vi "Day 10 - Pipe Maze.vi"() -> ()   [LabVIEW 2020, in "AoC 2023.lvlib"]
uses:
  AoC 2023.lvlib
  3d240fc5-b77a-4919-ab2e-2db28b4f468f.vi
  3d240fc5-b77a-4919-ab2e-2db28b4f468f.vi/a6c839c9-92fd-4c27-961e-592a9f44c727.vi
  <vilib>/Analysis/geometry.llb/Point in Polygon.vi
  <vilib>/Analysis/geometry.llb/Point in Polygon (Scalar).vi
panel:
  in  "Tab Control":enum32{"GRID", "CHART"}(tab)
  out "GRID":string[][](array[string])
  out "XY Graph":cluster{"X":dbl, "Y":dbl}[](graph)
  in  "TIMEOUT":i32
  out "Puzzle Part-2 Answer":string
  out "Puzzle Answer":string
  in  "Puzzle Inputs":string[](array[string])=["7-F7-\n.FJ|7\nSJLL7\n|F--J\nLJ.LJ", "-L|F7\n7S-7|\nL|7||\n-L-J|\nL|-JF", "7-F7-\n.FJ|7\nSJLL7\n|F--J\nLJ.LJ", "...........\n.S-------7.\n.|F-----7|.\n.||.....||.\n.||.....||.\n.|L-7.F-J|.\n.|..|.|..|.\n.L--J.L--J.\n...........", ".F----7F7F7F7F-7....\n.|F--7||||||||FJ....\n.||.FJ||||||||L7....\nFJL7L7LJLJ||LJ.L-7..\nL--J.L7...LJS7F-7L7.\n....F-J..F7FJ|L7L7L7\n....L7.F7||L7|.L7L7|\n.....|FJLJ|FJ|F7|.LJ\n....FJL-7.||.||||...\n....L---J.LJ.LJLJ...", "FF7FSF7F7F7F7F7F---7\nL|LJ||||||||||||F--J\nFL-7LJLJ||||||LJL-77\nF--JF--7||LJLJ7F7FJ-\nL---JF-JLJ.||-FJLJJ7\n|F|F-JF---7F7-L7L|7|\n|FFJF7L7F-JF7|JL---7\n7-L-JL7||F7|L7F-7F7|\nL.L7LFJ|||||FJL7||LJ\nL7JLJL-JLJLJL--JLJ.L"]
  # "Enter the Puzzle Input and run the VI"
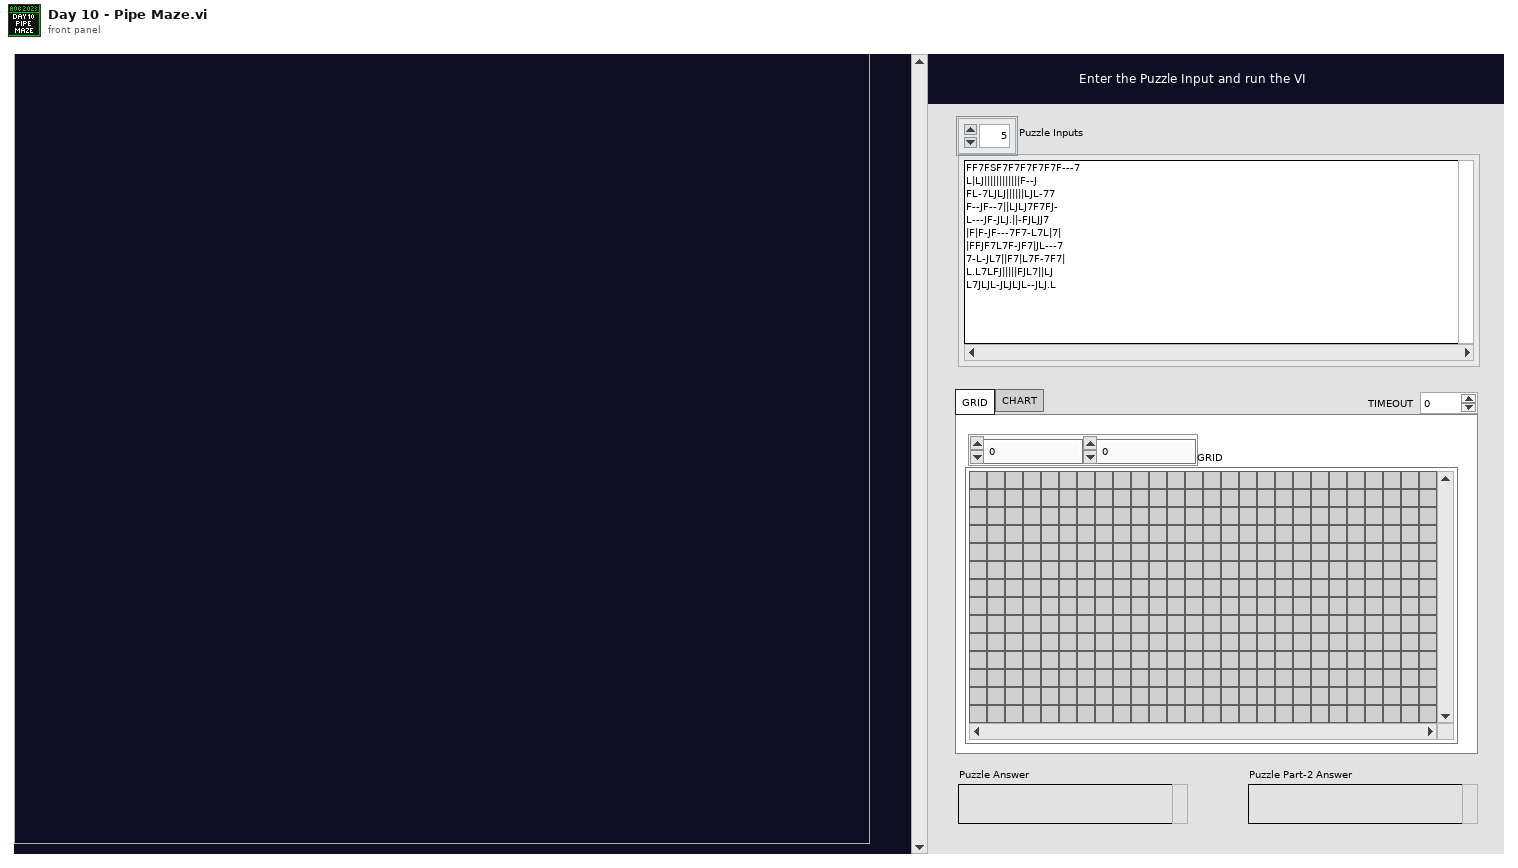
[diagram p1: front panel]
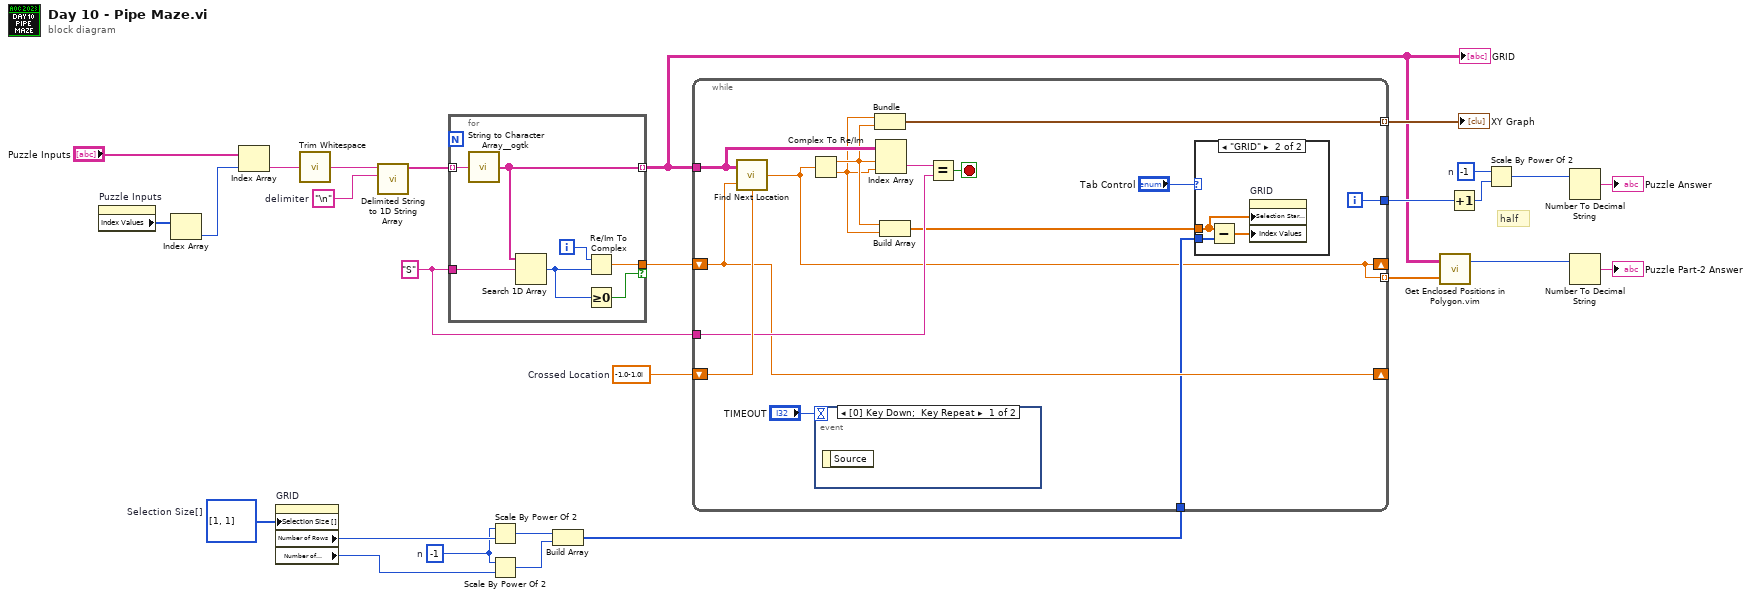
[diagram p0: block diagram]
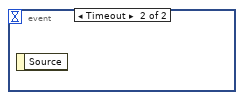
[diagram p3: hidden frame]
diagram:
  w9 = i16 -1  # n
  w11 = u32[] [1, 1]  # Selection Size[]
  w15 = i16 -1  # n
  w19 = cdb -1.0-1.0i  # Crossed Location
  w18 = "S"
  w25 = "\n"  # delimiter
  # "half"
  n1 = property on="Puzzle Inputs" class="Arr (strict)"() -> ("Index Values"=w13:u32[])  [unwired: 2 in, 2 out]
  n2 = Index Array(array=w13) -> (element=w12:u32)  [unwired: 1 in]
  n3 = Index Array(array="Puzzle Inputs", index=w12) -> (element=w21:string)
  n4 = property on="GRID" class="Arr (strict)"("Selection Size []"=w11) -> ("Number of Rows"=w10:u32, "Number of Columns"=w8:u32)  [unwired: 2 in, 2 out]
  n5 = call <vilib>:"Trim Whitespace.vi"("string"=w21) -> ("trimmed string"=w24:string)  [unwired: 1 in]
  n6 = call <vilib>:"Delimited String to 1D String Array.vi"("delimiter"=w25, "delimited string"=w24) -> ("string array"=w23:string[])  [unwired: 9 in]
  n7 = for {
    tunnel: w23 -> [w34] mode=indexing
    tunnel: [w33] -> w2 mode=indexing
    tunnel: w18 -> [w32]
    tunnel: [w29] -> w20 if=w28
    i -> [w31]
    n8 = call <userlib>:"String to Character Array__ogtk.vi"("Input String"=w34) -> ("Character Array"=w33:string[])
    n9 = Search 1D Array(1D array=w33, element=w32) -> (index of element=w30:i32)  [unwired: 1 in]
    n10 = Re/Im To Complex(1:w30, 2:w31) -> (0:w29:cdb)
    n11 = Greater Or Equal To 0?(x=w30) -> (x >= 0?=w28:bool)
  }
  "GRID" <- w2
  n12 = Scale By Power Of 2(n=w9, x=w10) -> (x*2^n=w6:u32)
  n13 = Scale By Power Of 2(n=w9, x=w8) -> (x*2^n=w7:u32)
  n14 = Build Array(w6, w7) -> (w5:u32[])
  n15 = while {
    tunnel: w2 -> [w48]
    tunnel: w18 -> [w46]
    tunnel: [w45] -> w17
    shift-right: [w44] -> _
    shift-left: w19 -> [w49]
    shift-right: [w36] -> _
    shift-left: w20 -> [w44]
    tunnel: w5 -> [w42]
    tunnel: [w38] -> w4 mode=indexing
    tunnel: [w36] -> w3 mode=indexing
    i -> [w45]
    stop <- w37 stop-if-true
    n16 = call "Find Next Location.vi"("Crossed Location"=w49, "Current Location"=w44, "Grid"=w48) -> ("Next Location"=w36:cdb)
    n17 = Complex To Re/Im(x + iy=w36) -> (x=w40:dbl, y=w39:dbl)
    n18 = event shown="[0] Key Down;  Key Repeat" {
      selector: _ -> [_ _]
      dyn-events: _ -> [_ _]
      timeout: "TIMEOUT" -> [_ _]
      event Key Down; Key Repeat {
        n19 = event-data() -> ()  [unwired: 1 in, 1 out]
      }
      event Timeout {
        n20 = event-data() -> ()  [unwired: 1 in, 1 out]
      }
    }
    n21 = Bundle(w39, w40) -> (w38:cluster{dbl, dbl})  [unwired: 1 in]
    n22 = Index Array(array=w48, index (row)=w40, index (col)=w39) -> (element=w47:string)
    n23 = Build Array(w40, w39) -> (w43:dbl[])
    n24 = Equal?(x=w47, y=w46) -> (x = y?=w37:bool)
    n25 = case shown="\"GRID\"" "Tab Control" {
      tunnel: w43 -> [_ w52]
      tunnel: w42 -> [_ w51]
      frame Default {
      }
      frame "GRID" {
        n26 = Subtract(x=w52, y=w51) -> (x-y=w50:dbl[])
        n27 = property on="GRID" class="Arr (strict)"("Selection Start []"=w52, "Index Values"=w50) -> ()  [unwired: 2 in, 2 out]
      }
    }
  }
  "XY Graph" <- w4
  n28 = call "Get Enclosed Positions in Polygon.vim"("Polygon"=w3, "2D Grid (for size)"=w2) -> ("#Enclosed Positions"=w1:u32)  [unwired: 1 out]
  n29 = Increment(x=w17) -> (x+1=w16:i32)
  n30 = Scale By Power Of 2(n=w15, x=w16) -> (x*2^n=w14:i32)
  n31 = Number To Decimal String(number=w14) -> (decimal integer string=→"Puzzle Answer":string)  [unwired: 1 in]
  n32 = Number To Decimal String(number=w1) -> (decimal integer string=→"Puzzle Part-2 Answer":string)  [unwired: 1 in]
